vi "read full data dictionary.vi"(8 "error in":errorcluster, 11 "data dictionary in":refnum<class "data dictionary.lvclass">) -> (0 "error out":errorcluster, 2 "dictionary":T1, 3 "data dictionary out":refnum<class "data dictionary.lvclass">)   [LabVIEW 2013, in "tag bus.lvlib" / "data dictionary.lvclass"]
doc: "Reads the entire data dictionary and returns it as a sorted set of tag names, organized by data type. This is very inefficient, duplicating the entire tag list and performing a sorting algorithm on this list."
uses:
  data dictionary.lvclass
  full data dictionary.ctl
  data dictionary.lvclass/data dictionary.ctl
  search/binary search.lvlib
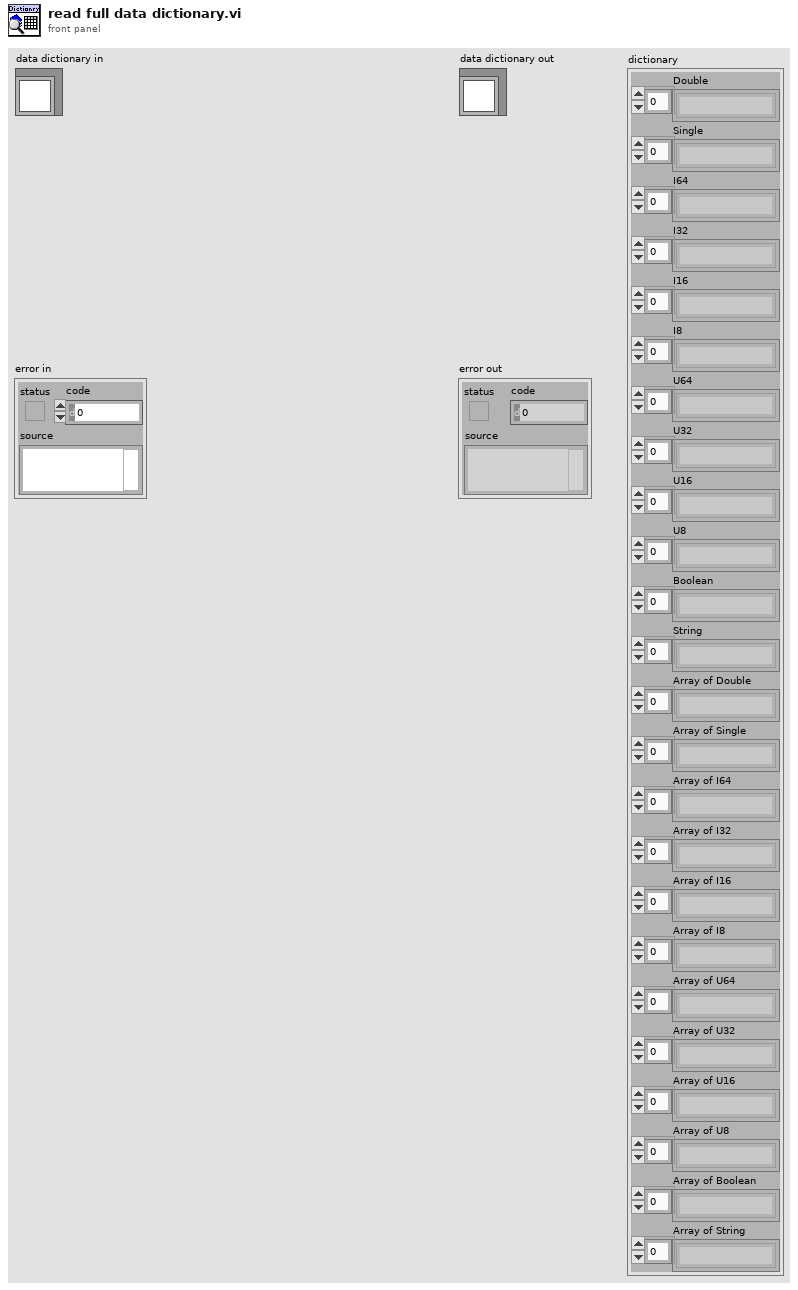
[diagram p1: front panel]
types:
  T1 = typedef "tag bus.lvlib/data dictionary.lvclass/full data dictionary.ctl" = cluster{"Double":string[], "Single":string[], "I64":string[], "I32":string[], "I16":string[], "I8":string[], "U64":string[], "U32":string[], "U16":string[], "U8":string[], "Boolean":string[], "String":string[], "Array of Double":string[], "Array of Single":string[], "Array of I64":string[], "Array of I32":string[], "Array of I16":string[], "Array of I8":string[], "Array of U64":string[], "Array of U32":string[], "Array of U16":string[], "Array of U8":string[], "Array of Boolean":string[], "Array of String":string[]}
  T2 = typedef "tag bus.lvlib/binary search.lvlib/sorted list.ctl" = cluster{"sorted strings":string[], "sorted indices":i32[]}
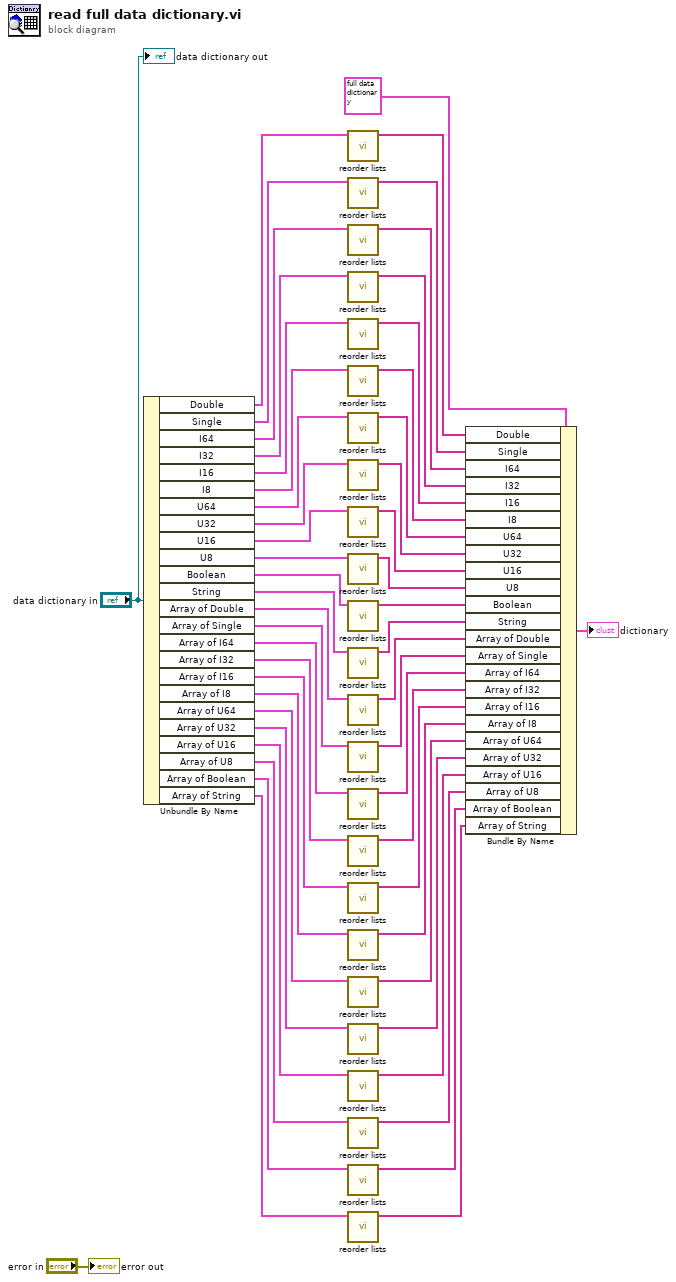
[diagram p0: block diagram]
diagram:
  n1 = Unbundle By Name("data dictionary in") -> ("Double"=w25:T2, "Single"=w48:T2, "I64"=w47:T2, "I32"=w46:T2, "I16"=w45:T2, "I8"=w44:T2, "U64"=w43:T2, "U32"=w42:T2, "U16"=w41:T2, "U8"=w40:T2, "Boolean"=w39:T2, "String"=w38:T2, "Array of Double"=w37:T2, "Array of Single"=w36:T2, "Array of I64"=w35:T2, "Array of I32"=w34:T2, "Array of I16"=w32:T2, "Array of I8"=w33:T2, "Array of U64"=w31:T2, "Array of U32"=w30:T2, "Array of U16"=w29:T2, "Array of U8"=w28:T2, "Array of Boolean"=w27:T2, "Array of String"=w26:T2)
  n2 = call "reorder lists.vi"("sorted list"=w25) -> ("ordered list"=w24:string[])  [unwired: 10 in]
  n3 = call "reorder lists.vi"("sorted list"=w48) -> ("ordered list"=w23:string[])  [unwired: 10 in]
  n4 = call "reorder lists.vi"("sorted list"=w47) -> ("ordered list"=w1:string[])  [unwired: 10 in]
  n5 = call "reorder lists.vi"("sorted list"=w46) -> ("ordered list"=w2:string[])  [unwired: 10 in]
  n6 = call "reorder lists.vi"("sorted list"=w45) -> ("ordered list"=w3:string[])  [unwired: 10 in]
  n7 = call "reorder lists.vi"("sorted list"=w44) -> ("ordered list"=w4:string[])  [unwired: 10 in]
  n8 = call "reorder lists.vi"("sorted list"=w43) -> ("ordered list"=w5:string[])  [unwired: 10 in]
  n9 = call "reorder lists.vi"("sorted list"=w42) -> ("ordered list"=w6:string[])  [unwired: 10 in]
  n10 = call "reorder lists.vi"("sorted list"=w41) -> ("ordered list"=w7:string[])  [unwired: 10 in]
  n11 = call "reorder lists.vi"("sorted list"=w40) -> ("ordered list"=w8:string[])  [unwired: 10 in]
  n12 = call "reorder lists.vi"("sorted list"=w39) -> ("ordered list"=w9:string[])  [unwired: 10 in]
  n13 = call "reorder lists.vi"("sorted list"=w38) -> ("ordered list"=w10:string[])  [unwired: 10 in]
  n14 = call "reorder lists.vi"("sorted list"=w37) -> ("ordered list"=w11:string[])  [unwired: 10 in]
  n15 = call "reorder lists.vi"("sorted list"=w36) -> ("ordered list"=w12:string[])  [unwired: 10 in]
  n16 = call "reorder lists.vi"("sorted list"=w35) -> ("ordered list"=w13:string[])  [unwired: 10 in]
  n17 = call "reorder lists.vi"("sorted list"=w34) -> ("ordered list"=w14:string[])  [unwired: 10 in]
  n18 = call "reorder lists.vi"("sorted list"=w32) -> ("ordered list"=w16:string[])  [unwired: 10 in]
  n19 = call "reorder lists.vi"("sorted list"=w33) -> ("ordered list"=w15:string[])  [unwired: 10 in]
  n20 = call "reorder lists.vi"("sorted list"=w31) -> ("ordered list"=w17:string[])  [unwired: 10 in]
  n21 = call "reorder lists.vi"("sorted list"=w30) -> ("ordered list"=w18:string[])  [unwired: 10 in]
  n22 = call "reorder lists.vi"("sorted list"=w29) -> ("ordered list"=w19:string[])  [unwired: 10 in]
  n23 = call "reorder lists.vi"("sorted list"=w28) -> ("ordered list"=w20:string[])  [unwired: 10 in]
  n24 = call "reorder lists.vi"("sorted list"=w27) -> ("ordered list"=w21:string[])  [unwired: 10 in]
  n25 = call "reorder lists.vi"("sorted list"=w26) -> ("ordered list"=w22:string[])  [unwired: 10 in]
  n26 = Bundle By Name(cluster=T1 {"Double"=[], "Single"=[], "I64"=[], "I32"=[], "I16"=[], "I8"=[], "U64"=[], "U32"=[], "U16"=[], "U8"=[], "Boolean"=[], "String"=[], "Array of Double"=[], "Array of Single"=[], "Array of I64"=[], "Array of I32"=[], "Array of I16"=[], "Array of I8"=[], "Array of U64"=[], "Array of U32"=[], "Array of U16"=[], "Array of U8"=[], "Array of Boolean"=[], "Array of String"=[]} ("dictionary"), "Double"=w24, "Single"=w23, "I64"=w1, "I32"=w2, "I16"=w3, "I8"=w4, "U64"=w5, "U32"=w6, "U16"=w7, "U8"=w8, "Boolean"=w9, "String"=w10, "Array of Double"=w11, "Array of Single"=w12, "Array of I64"=w13, "Array of I32"=w14, "Array of I16"=w16, "Array of I8"=w15, "Array of U64"=w17, "Array of U32"=w18, "Array of U16"=w19, "Array of U8"=w20, "Array of Boolean"=w21, "Array of String"=w22) -> (→"dictionary":T1)
  "error out" <- "error in"
  "data dictionary out" <- "data dictionary in"
